vi "mecanum tank 1.vi"   [LabVIEW 2012, in "Mecanum Drive.lvrbt"]
uses:
  Mecanum Drive.lvrbt
  <vilib>/NXT/Hardware/Plugins/Tetrix 180 deg Servo/Tetrix180ServoAddress.ctl
  <vilib>/NXT/Hardware/Plugins/Tetrix DC Motor/TetrixDCMotorAddress.ctl
  <vilib>/NXT/NXTIO Xnodes/NXTIONodeSubVIs/TETRIX IO Move Servos.vi
  <vilib>/NXT/NXTIO Xnodes/NXTIONodeSubVIs/TETRIX IO Move DC Motors.vi
  <vilib>/NXT/Dual Mode Library/Display/drawNumber.vi
  <vilib>/NXT/NXTIO Xnodes/NXTIONodeSubVIs/TETRIX IO Check Battery.vi
  <vilib>/NXT/NXTIO Xnodes/NXTIONodeSubVIs/TETRIX IO Stop DC Motors.vi
  <vilib>/NXT/NXTIO Xnodes/AddressXNode/NXTIOAddress.xnode
  <vilib>/NXT/Subs/LVHSConnector.ctl
  <vilib>/NXT/NXTIO Xnodes/NXTIOXNode/NXTIO.xnode
  <vilib>/NXT/LegoClasses/BrickReference/BrickReference.lvclass
panel:
  # "This VI was generated based on your configuration in the Remote Control Editor. You may modify the code as needed for your robot. To test this program for an FTC match, return to the Remote Control Editor, select the \"Run Program\" tab, and choose \"Teleop\"."
types:
  T1 = typedef "Tetrix180ServoAddress.ctl" = i32
  T2 = typedef "TetrixDCMotorAddress.ctl" = i32
  T3 = cluster{"TetrixDCMotor":T2, "TetrixDCMotor 2":T2}
  T4 = typedef "LVHSConnector.ctl" = refnum<class "BrickReference.lvclass">
  T5 = typedef "FTC ControllerState.ctl" = cluster{"Left X":i8, "Left Y":i8, "Right X":i8, "Right Y":i8, "Button Encoding 9-12":u8, "Button Encoding 1-8":u8, "POV":T6}
  T6 = typedef "FTC POVState.ctl" = i8
  T7 = typedef "FTC ButtonEventType.ctl" = enum16{"Pressed", "Released"}
  T8 = cluster{"Button ID":enum16{"None", "Button 1", "Button 2", "Button 3", "Button 4", "Button 5", "Button 6", "Button 7", "Button 8", "Button 9", "Button 10", "Button 11", "Button 12", "POV Up", "POV Up Right", "POV Right", "POV Down Right", "POV Down", "POV Down Left", "POV Left", "POV Up Left"}, "Event Type":T7}[]
  T9 = typedef "FTC ButtonState.ctl" = cluster{"Button 1":bool, "Button 2":bool, "Button 3":bool, "Button 4":bool, "Button 5":bool, "Button 6":bool, "Button 7":bool, "Button 8":bool, "Button 9":bool, "Button 10":bool, "Button 11":bool, "Button 12":bool, "POV":T6}
  T10 = enum16{"None", "Button 1", "Button 2", "Button 3", "Button 4", "Button 5", "Button 6", "Button 7", "Button 8", "Button 9", "Button 10", "Button 11", "Button 12", "POV Up", "POV Up Right", "POV Right", "POV Down Right", "POV Down", "POV Down Left", "POV Left", "POV Up Left"}
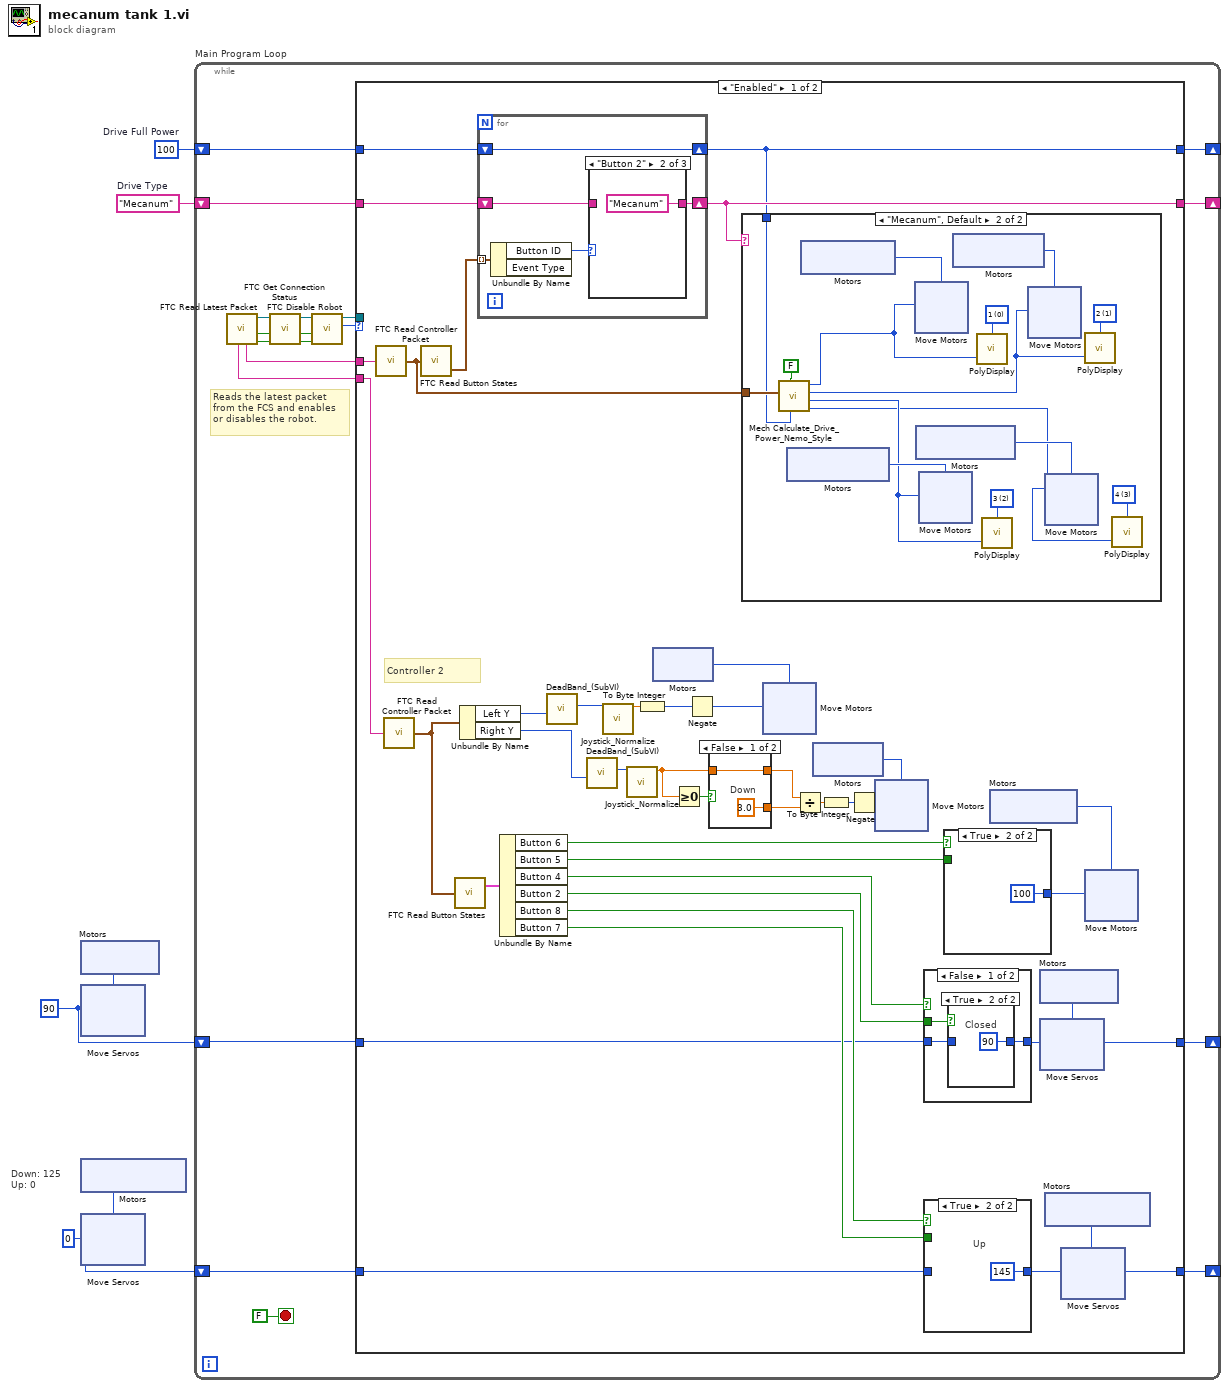
[diagram p0: block diagram]
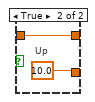
[diagram p2: hidden frame]
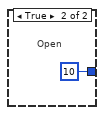
[diagram p4: hidden frame]
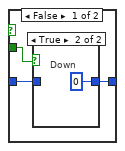
[diagram p5: hidden frame]
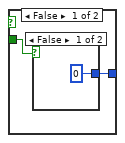
[diagram p7: hidden frame]
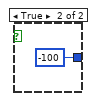
[diagram p8: hidden frame]
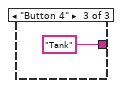
[diagram p11: hidden frame]
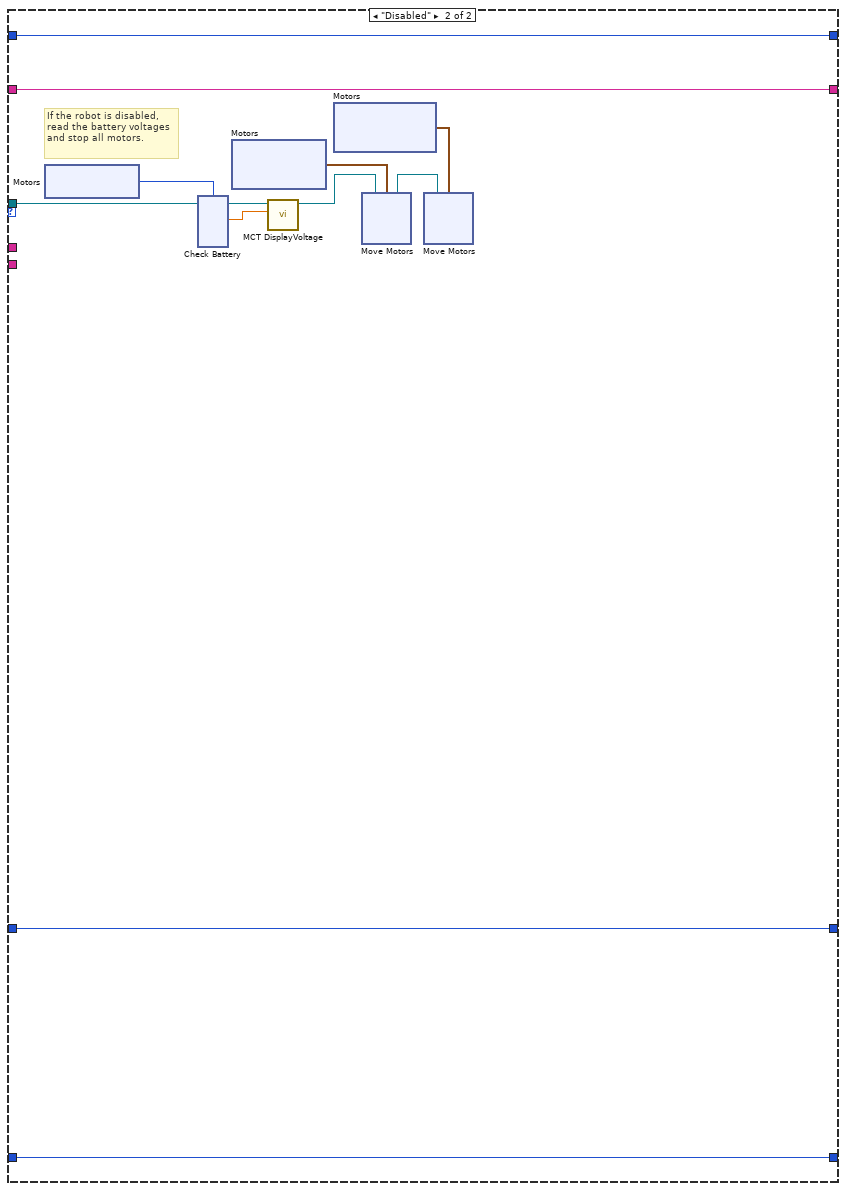
[diagram p12: hidden frame]
diagram:
  w1 = u8 0 ("Position 1")
  w3 = u8 90 ("Position 1")
  w5 = 100  # Drive Full Power
  w6 = "Mecanum"  # Drive Type
  # "Down: 125\nUp: 0"
  n1 = xnode "Motors"() -> ("Motor"=w4:T1)
  n2 = xnode "Move Servos"("Position 1"=w3, "Motors"=w4) -> ()  [unwired: 1 in, 1 out]
  n3 = xnode "Motors"() -> ("Motor"=w2:T1)
  n4 = xnode "Move Servos"("Position 1"=w1, "Motors"=w2) -> ()  [unwired: 1 in, 1 out]
  n5 = while "Main Program Loop" {
    shift-right: [w13] -> _
    shift-left: w6 -> [w14]
    shift-right: [w11] -> _
    shift-left: w5 -> [w12]
    shift-right: [w9] -> _
    shift-left: w3 -> [w10]
    shift-right: [w7] -> _
    shift-left: w1 -> [w8]
    stop <- FALSE stop-if-true
    # "Reads the latest packet\nfrom the FCS and enables\nor disables the robot."
    n6 = call <vilib>:"FTC Read Latest Packet.vi"() -> ("Packet Received?"=w22:bool, "Stopped?"=w19:bool, "NXT"=w21:T4, "Controller 1"=w24:string, "Controller 2"=w23:string)  [unwired: 6 in, 1 out]
    n7 = call <vilib>:"FTC Get Connection Status.vi"("Packet Received?"=w22, "Stopped?"=w19, "NXT"=w21) -> ("Online?"=w16:bool, "Stopped?"=w17:bool, "NXT"=w18:T4)  [unwired: 5 in]
    n8 = call <vilib>:"FTC Disable Robot.vi"("Online?"=w16, "Stopped?"=w17, "NXT"=w18) -> ("Enabled?"=w20:enum16{"Disabled", "Enabled"}, "NXT"=w15:T4)  [unwired: 3 in]
    n9 = case "disableCase" shown="\"Enabled\"" w20 {
      tunnel: w24 -> [w65 _]
      tunnel: w23 -> [w64 _]
      tunnel: w15 -> [_ w193]
      tunnel: w14 -> [w62 w185]
      tunnel: [w61 w185] -> w13
      tunnel: w12 -> [w59 w184]
      tunnel: [w58 w184] -> w11
      tunnel: w10 -> [w34 w183]
      tunnel: [w37 w183] -> w9
      tunnel: w8 -> [w39 w182]
      tunnel: [w42 w182] -> w7
      frame "Enabled" {
        # "Controller 2"
        n10 = call <vilib>:"FTC Read Controller Packet.vi"("Packet"=w65) -> ("Controller State"=w60:T5)  [unwired: 4 in]
        n11 = call <vilib>:"FTC Read Controller Packet.vi"("Packet"=w64) -> ("Controller State"=w51:T5)  [unwired: 4 in]
        n12 = call <vilib>:"FTC Read Button States.vi"("Controller State"=w60) -> ("Button Events"=w63:T8)  [unwired: 2 in, 1 out]
        n13 = call <vilib>:"FTC Read Button States.vi"("Controller State"=w51) -> ("Button States"=w50:T9)  [unwired: 2 in, 1 out]
        n14 = Unbundle By Name(w51) -> ("Left Y"=w57:i8, "Right Y"=w52:i8)
        n15 = for {
          tunnel: w63 -> [w178] mode=indexing
          shift-right: [w176] -> w61
          shift-left: w62 -> [w175]
          shift-right: [w174] -> w58
          shift-left: w59 -> [w174]
          n16 = Unbundle By Name(w178) -> ("Button ID"=w177:T10)  [unwired: 1 out]
          n17 = case shown="\"Button 2\"" w177 {
            tunnel: [w179 "Mecanum" "Tank"] -> w176
            tunnel: w175 -> [w179 _ _]
            frame "None", Default {
            }
            frame "Button 2" {
            }
            frame "Button 4" {
            }
          }
        }
        n18 = Unbundle By Name(w50) -> ("Button 6"=w47:bool, "Button 5"=w46:bool, "Button 4"=w35:bool, "Button 2"=w36:bool, "Button 8"=w41:bool, "Button 7"=w40:bool)
        n19 = call "DeadBand_(SubVI).vi"("Axis In"=w57) -> ("Axis out"=w56:i8)  [unwired: 10 in]
        n20 = call "DeadBand_(SubVI).vi"("Axis In"=w52) -> ("Axis out"=w53:i8)  [unwired: 10 in]
        n21 = call "Joystick_Normalize.vi"("Joystick In"=w56) -> ("Norm Out"=w55:sgl)  [unwired: 10 in]
        n22 = call "Joystick_Normalize.vi"("Joystick In"=w53) -> ("Norm Out"=w28:sgl)  [unwired: 10 in]
        n23 = To Byte Integer(number=w55) -> (8bit integer=w31:i8)
        n24 = xnode "Motors"() -> ("Motor"=w54:T2)
        n25 = Greater Or Equal To 0?(x=w28) -> (x >= 0?=w29:bool)
        n26 = Negate(x=w31) -> (-x=w30:i8)
        n27 = case shown="False" w29 {
          tunnel: [w67 w69] -> w26
          tunnel: w28 -> [w67 w69]
          tunnel: [3.0 10.0] -> w27
          frame False {
            # "Down"
          }
          frame True {
            # "Up"
          }
        }
        n28 = case shown="\"Mecanum\", Default" w61 {
          tunnel: w60 -> [_ w129]
          tunnel: w58 -> [_ w127]
          frame "Tank" {
          }
          frame "Mecanum", Default {
            w131 = i16 3 items=["1", "2", "3", "4", "5", "6", "7", "8", "9", "10", "11", "12"] ("Line")
            w133 = i16 2 items=["1", "2", "3", "4", "5", "6", "7", "8", "9", "10", "11", "12"] ("Line")
            w135 = i16 1 items=["1", "2", "3", "4", "5", "6", "7", "8", "9", "10", "11", "12"] ("Line")
            w136 = i16 0 items=["1", "2", "3", "4", "5", "6", "7", "8", "9", "10", "11", "12"] ("Line")
            n29 = call "Mech Calculate_Drive_Power_Nemo_Style.vi"("Power"=w127, "Reverse"=FALSE, "Controller State"=w129) -> ("Right Rear Power"=w130:i8, "Right Front Power"=w132:i8, "Left Rear Power"=w134:i8, "Left Front Power"=w128:i8)  [unwired: 5 in]
            n30 = xnode ("Motors")() -> ("Motor"=w141:T2)
            n31 = xnode ("Motors")() -> ("Motor"=w138:T2)
            n32 = xnode ("Move Motors")("Power/Speed 1"=w128, "Motors"=w138) -> ()  [unwired: 1 in, 1 out]
            n33 = xnode ("Motors")() -> ("Motor"=w140:T2)
            n34 = xnode ("Move Motors")("Power/Speed 1"=w132, "Motors"=w141) -> ()  [unwired: 1 in, 1 out]
            n35 = xnode ("Motors")() -> ("Motor"=w139:T2)
            n36 = call-poly <vilib>:"PolyDisplay.vi"("number"=w128, "Line"=w136) -> ()  [unwired: 2 in, 1 out]
            n37 = call-poly <vilib>:"PolyDisplay.vi"("number"=w132, "Line"=w133) -> ()  [unwired: 2 in, 1 out]
            n38 = xnode ("Move Motors")("Power/Speed 1"=w134, "Motors"=w139) -> ()  [unwired: 1 in, 1 out]
            n39 = xnode ("Move Motors")("Power/Speed 1"=w130, "Motors"=w140) -> ()  [unwired: 1 in, 1 out]
            n40 = call-poly <vilib>:"PolyDisplay.vi"("number"=w134, "Line"=w135) -> ()  [unwired: 2 in, 1 out]
            n41 = call-poly <vilib>:"PolyDisplay.vi"("number"=w130, "Line"=w131) -> ()  [unwired: 2 in, 1 out]
          }
        }
        n42 = xnode "Move Motors"("Power/Speed 1"=w30, "Motors"=w54) -> ()  [unwired: 1 in, 1 out]
        n43 = Divide(x=w26, y=w27) -> (x/y=w32:dbl)
        n44 = xnode "Motors"() -> ("Motor"=w49:T2)
        n45 = To Byte Integer(number=w32) -> (8bit integer=w48:i8)
        n46 = Negate(x=w48) -> (-x=w33:i8)
        n47 = xnode "Move Motors"("Power/Speed 1"=w33, "Motors"=w49) -> ()  [unwired: 1 in, 1 out]
        n48 = case shown="False" w35 {
          tunnel: w36 -> [w72 _]
          tunnel: [w71 u8 10] -> w37
          tunnel: w34 -> [w70 _]
          frame False {
            n49 = case shown="True" w72 {
              tunnel: [w73 u8 90] -> w71
              tunnel: w70 -> [w73 _]
              frame False {
              }
              frame True {
                # "Closed"
              }
            }
          }
          frame True {
            # "Open"
          }
        }
        n50 = case shown="True" w41 {
          tunnel: w40 -> [w86 _]
          tunnel: [w85 u8 145] -> w42
          tunnel: w39 -> [w84 _]
          frame False {
            n51 = case shown="True" w86 {
              tunnel: [w87 u8 0] -> w85
              tunnel: w84 -> [w87 _]
              frame False {
              }
              frame True {
                # "Down"
              }
            }
          }
          frame True {
            # "Up"
          }
        }
        n52 = case shown="True" w47 {
          tunnel: w46 -> [w107 _]
          tunnel: [w106 i8 100] -> w44
          frame False {
            n53 = case shown="False" w107 {
              tunnel: [i8 0 i8 -100] -> w106
              frame False {
              }
              frame True {
              }
            }
          }
          frame True {
          }
        }
        n54 = xnode "Motors"() -> ("Motor"=w45:T2)
        n55 = xnode "Motors"() -> ("Motor"=w38:T1)
        n56 = xnode "Move Servos"("Position 1"=w37, "Motors"=w38) -> ()  [unwired: 1 in, 1 out]
        n57 = xnode "Motors"() -> ("Motor"=w43:T1)
        n58 = xnode "Move Servos"("Position 1"=w42, "Motors"=w43) -> ()  [unwired: 1 in, 1 out]
        n59 = xnode "Move Motors"("Power/Speed 1"=w44, "Motors"=w45) -> ()  [unwired: 1 in, 1 out]
      }
      frame "Disabled" {
        # "If the robot is disabled, read the battery voltages and stop all motors."
        n60 = xnode ("Motors")() -> ("Motor"=w192:T2)
        n61 = xnode ("Check Battery")("Motors"=w192, "NXT/EV3"=w193) -> ("Voltage 1"=w191:sgl, "NXT/EV3"=w190:T4)
        n62 = xnode "Motors"() -> ("Motor"=w189:cluster{"TetrixDCMotor":T2, "TetrixDCMotor":T2})
        n63 = call <vilib>:"MCT DisplayVoltage.vi"("Motor Voltage"=w191, "NXT"=w190) -> ("NXT"=w188:T4)  [unwired: 9 in]
        n64 = xnode "Motors"() -> ("Motor"=w187:cluster{"TetrixDCMotor":T2, "TetrixDCMotor":T2})
        n65 = xnode "Move Motors"("Motors"=w189, "NXT/EV3"=w188) -> ("NXT/EV3"=w186:T4)
        n66 = xnode "Move Motors"("Motors"=w187, "NXT/EV3"=w186) -> ()  [unwired: 1 out]
      }
    }
  }
